vi "demo_GLA Summit.vi"(11 "Stop Demo":refnum<user-event>) -> ()   [LabVIEW 2020]
panel:
  # "GLA Summit is a worldwide 24-hour onslaught of LabVIEW presentations from around the globe\n\nWelcome for advanced LabVIEW developers and Architects (certified or self-proclaimed) from around the world to network and participate in an inclusive, all-digital, free event.\nhttps://www.glasummit.org/\nhttps://events.ringcentral.com/events/gla-summit-2025"
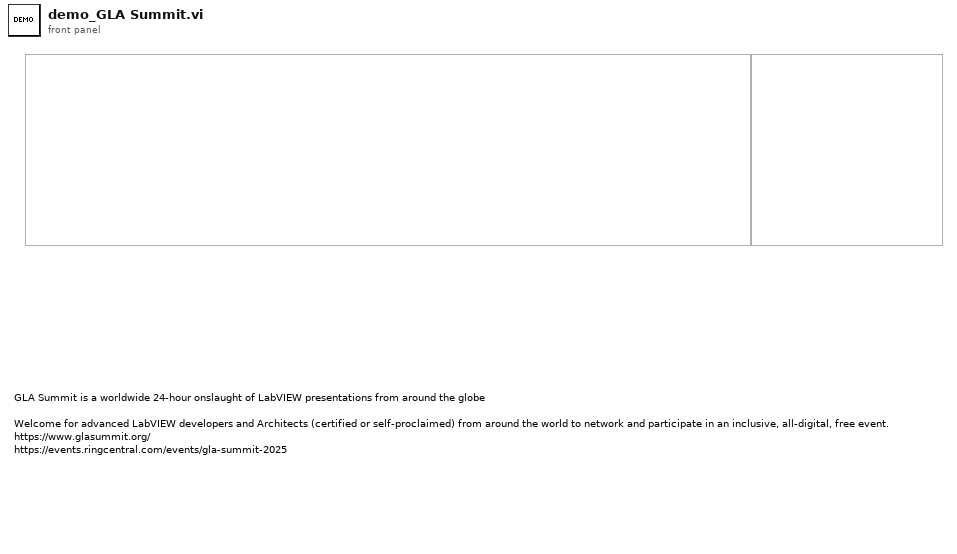
[diagram p1: front panel]
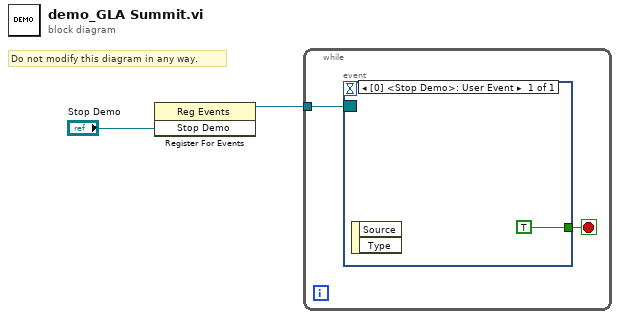
[diagram p0: block diagram]
diagram:
  # "Do not modify this diagram in any way."
  n1 = register-events("Stop Demo") -> (reference out=w1:refnum<event-registration>)  [unwired: 2 in, 1 out]
  n2 = while {
    tunnel: w1 -> [w4]
    stop <- w3 stop-if-true
    n3 = event shown="[0] <Stop Demo>: User Event" {
      selector: w4 -> [_]
      dyn-events: _ -> [_]
      timeout: _ -> [_]
      tunnel: [TRUE] -> w3
      event User Event {
        n4 = event-data() -> ()  [unwired: 1 in, 2 out]
      }
    }
  }
